vi "RSZVB Get Signal Source.vi"(8 "error in (no error)":errorcluster {"code" format="%.0x"}, 9 "Stage (1)":i32=1, 10 "Channel (1)":i32=1, 11 "VISA resource name":refnum<visa-resource-name>) -> (0 "error out":errorcluster {"code" format="%.0x"}, 1 "Port Number":i32, 2 "Source":i32, 3 "VISA resource name out":refnum<visa-resource-name>)   [LabVIEW 2011]
doc: "This VI returns an analyzer or an external generator port as a signal source for the LO 1 or L0 2 signal.\n\nRemote-control command(s):\n[SENSe<Ch>:]FREQuency:CONVersion:MIXer:LOPort<Stg>?"
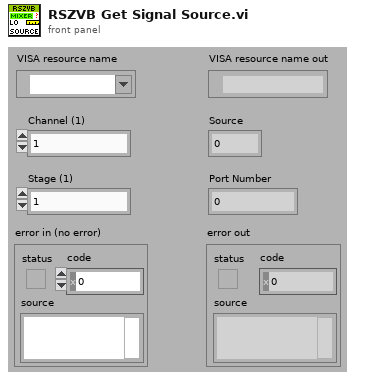
[diagram p1: front panel]
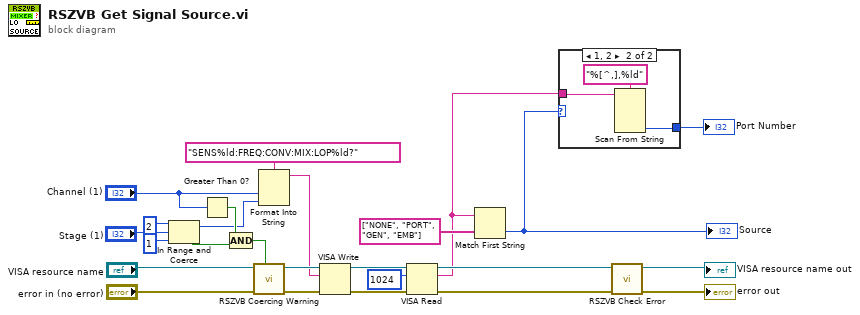
[diagram p0: block diagram]
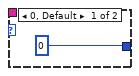
[diagram p2: hidden frame]
diagram:
  n1 = In Range and Coerce(upper limit=2, x="Stage (1)", lower limit=1) -> (coerced(x)=w7:i32, In Range?=w11:bool)
  n2 = Greater Than 0?(x="Channel (1)") -> (x > 0?=w8:bool)
  n3 = Compound Arithmetic op=AND(w8, w11) -> (w9:bool)
  n4 = call "RSZVB Coercing Warning.vi"("In Range?"=w9, "error in (no error)"="error in (no error)", "VISA session"="VISA resource name") -> ("error out"=w24:errorcluster, "dup VISA session"=w25:refnum<visa-resource-name>)  [unwired: 7 in]
  n5 = Format Into String(format string="SENS%ld:FREQ:CONV:MIX:LOP%ld?", "Channel (1)", w7) -> (resulting string=w17:string)  [unwired: 2 in, 1 out]
  n6 = VISA Write(VISA resource name=w25, write buffer=w17, error in (no error)=w24) -> (VISA resource name out=w21:refnum<visa-resource-name>, error out=w22:errorcluster)  [unwired: 1 out]
  n7 = VISA Read(VISA resource name=w21, byte count=u32 1024 ("byte count (0)"), error in (no error)=w22) -> (VISA resource name out=w19:refnum<visa-resource-name>, read buffer=w2:string, error out=w20:errorcluster)  [unwired: 1 out]
  n8 = Match First String(2:string[] ["NONE", "PORT", "GEN", "EMB"], 3:w2) -> (0:w1:i32)  [unwired: 1 out]
  "Source" <- w1
  n9 = case shown="1, 2" w1 {
    tunnel: w2 -> [_ w28]
    tunnel: [0 w27] -> w4
    frame 0, Default {
    }
    frame 1, 2 {
      n10 = Scan From String(format string="%[^,],%ld", input string=w28) -> (output 2=w27:i32)  [unwired: 5 in, 3 out]
    }
  }
  "Port Number" <- w4
  n11 = call "RSZVB Check Error.vi"("error in (no error)"=w20, "VISA session"=w19) -> ("error out"=→"error out":errorcluster, "dup VISA session"=→"VISA resource name out":refnum<visa-resource-name>)  [unwired: 8 in]
